vi "Shooter Loop.vi"(11 "Shooter Control":T2) -> (0 "Punch":T1, 1 "Trigger":T1, 2 "Release":T1, 3 "Add":T1, 5 "State":T4, 7 "Is Ready?":bool)   [LabVIEW 2013]
uses:
  <vilib>/Rock Robotics/WPI/Solenoid/WPI_SolenoidValue.ctl
  Common Code/Shooter State.ctl
  Shooter Manual Control.ctl
  Shooter Command.ctl
  Shooter Status.ctl
  Common Code/Change Detect Int.vi
  Common Code/Change Detect Boolean.vi
  Robot Global Data.vi
  <vilib>/Rock Robotics/WPI/DigitalInput/WPI_DigitalInputRefNum Registry Get.vi
  <vilib>/Rock Robotics/WPI/DigitalInput/WPI_DigitalInputGetValue.vi
panel:
  in  "Is Retracted":bool
  in  "Pressure":dbl
  in  "Line":dbl
  in  "Reset Time":dbl
  in  "Release Time":dbl
  # "Debug controls under this box"
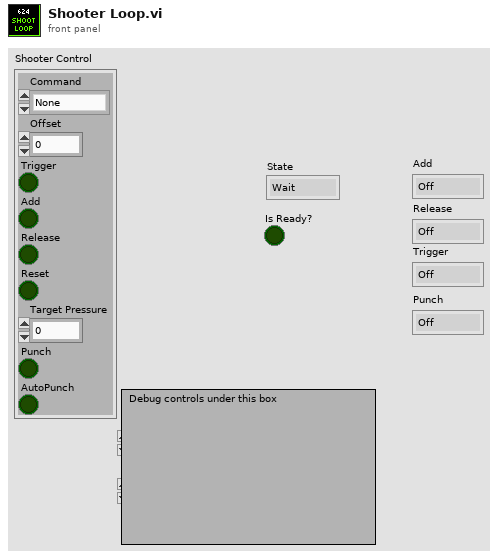
[diagram p1: front panel]
types:
  T1 = typedef "WPI_SolenoidValue.ctl" = enum16{"Off", "On", "Forward", "Reverse"}
  T2 = typedef "Shooter Manual Control.ctl" = cluster{"Command":T3, "Offset":dbl, "Trigger":bool, "Add":bool, "Release":bool, "Reset":bool, "Target Pressure":dbl, "Punch":bool, "AutoPunch":bool}
  T3 = typedef "Shooter Command.ctl" = enum16{"None", "Warmup", "Shoot", "Line Shoot", "Soft Shoot", "Toss"}
  T4 = typedef "Shooter State.ctl" = enum16{"Wait", "Fill Piston", "Lift Halo", "Trigger", "Reset", "Soft Release", "Soft Unpin", "Soft Refill", "Soft Shoot", "Toss Prep", "Toss Release"}
  T5 = typedef "Shooter Status.ctl" = cluster{"Shooter Ready":bool, "Add":bool, "Punch":bool, "Release":bool, "Trigger":bool, "High":bool, "State":T4}
  T6 = typedef "Dashboard UDP Packet.ctl" = cluster{"Camera":T7, "Gyro":T8, "Encoder":T10, "Auto Shift":T11, "Auton":T12, "Drive/Ramp X":dbl, "Drive/Ramp Y":dbl, "Drive/Battery Cutoff":dbl, "Pressure/Compressor Min Voltage":dbl, "Pressure/Compressor Delay":dbl, "Controller/Strafe Correction":bool, "Shooter":T13, "Rollers":T14, "Abort":bool, "Finish":bool, "IR Halo Sustain Time":dbl, "Disable Compressor":bool, "Center Omni Drive Delay":i32, "Vision Mode":T15, "Radius Throttle":bool, "Fieldcentric":T16, "Roll":T17, "Stick Deadband":dbl}
  T7 = typedef "Camera Controls.ctl" = cluster{"Camera/View Angle X":dbl, "Camera/Goal Track Timeout":dbl, "Camera/View Angle Y":dbl, "Camera/Goal Exposure":dbl, "Camera/Vision Receive Timeout":dbl, "Camera/Offset 1":dbl, "Camera/Offset 2":dbl}
  T8 = typedef "Gyro Controls.ctl" = cluster{"Gyro/Angle Tolerance":dbl, "Gyro/Steer Closeness Threshold":dbl, "Steer PID":T9, "Steer Close PID":T9}
  T9 = typedef "PID Params.ctl" = cluster{"max":dbl, "min":dbl, "P":dbl, "I":dbl, "D":dbl}
  T10 = typedef "Encoder Controls.ctl" = cluster{"Encoders/Reset":bool, "Encoders/Omni Constant":dbl, "Encoders/Omni Tick Constant":dbl, "Encoders/Left Constant":dbl, "Encoders/Right Constant":dbl, "Encoders/Right Tick Constant":dbl}
  T11 = typedef "Auto Shift Controls.ctl" = cluster{"AutoShift/Upshift Throttle Accel":dbl, "AutoShift/Speed Threshold":dbl, "AutoShift/Upshift Throttle":dbl, "AutoShift/Upshift Accel":dbl, "AutoShift/Downshift Accel":dbl, "AutoShift/Downshift Throttle":dbl, "AutoShift/Delay":dbl, "AutoShift/Enabled":bool}
  T12 = typedef "Auton Controls.ctl" = cluster{"Auton/Left Shoot X-Coord":dbl, "Auton/Right Shoot X-Coord":dbl, "DistDrive/Distance Stop Threshold":dbl, "DistDrive/Max Stop Speed":dbl, "Auton/Back Piston Time":dbl, "Auton/Manual Hot":bool, "Auton/Manual Hot Right":bool, "Default X PID":T9, "Default Y PID":T9, "Half Over Delay":dbl}
  T13 = typedef "Shooter Controls.ctl" = cluster{"Shooter/Reset Time":dbl, "Shooter/Release Delay":dbl, "Shooter/Pressure Steady Time":dbl, "Shooter/Misfire Delay":dbl, "Shooter/Ball Settle Time":dbl, "Shooter/Line IR Delay":dbl, "Pressure/Upper PSI Time":dbl, "Pressure/Lower PSI Time":dbl, "Shooter/Punch Delay":dbl, "Shooter/Target Pressure":dbl, "Pressure/Line B":dbl, "Pressure/Line M":dbl, "Pressure/Shooter M":dbl, "Pressure/Shooter B":dbl, "Halo Time":dbl, "Soft Release Delay":dbl, "Soft Unpin Delay":dbl, "Soft Shoot Delay":dbl, "Toss Release Time":dbl}
  T14 = typedef "Roller Controls.ctl" = cluster{"Roller/Load IRs Verify Time":dbl, "Roller/Center IR Latch Time":dbl, "Roller/Speed Front":dbl, "Roller/Speed Back":dbl, "Roller/Entry Timeout":dbl, "Roller/To Center Timeout":dbl, "Roller/Sustain Time":dbl, "Roller/Verify Center Time":dbl}
  T15 = typedef "Vision Mode.ctl" = enum16{"Normal", "Extreme Left", "Extreme Right"}
  T16 = typedef "Fieldcentric Controls.ctl" = cluster{"Relative Angle":bool, "Point Robot":bool, "X/Y ratio low":dbl, "Steering Gain":dbl, "Force Omni Down":bool, "Enable":bool, "X/Y ratio high":dbl}
  T17 = typedef "Roll Maneuver.ctl" = cluster{"X 1":dbl, "Y 1":dbl, "Y 2":dbl, "X 2":dbl, "Y 3":dbl, "X 3":dbl, "Time 1":i32, "Time 2":i32, "Time 3":i32, "Angle Start":dbl, "Angle End":dbl, "Angle Linearity":dbl}
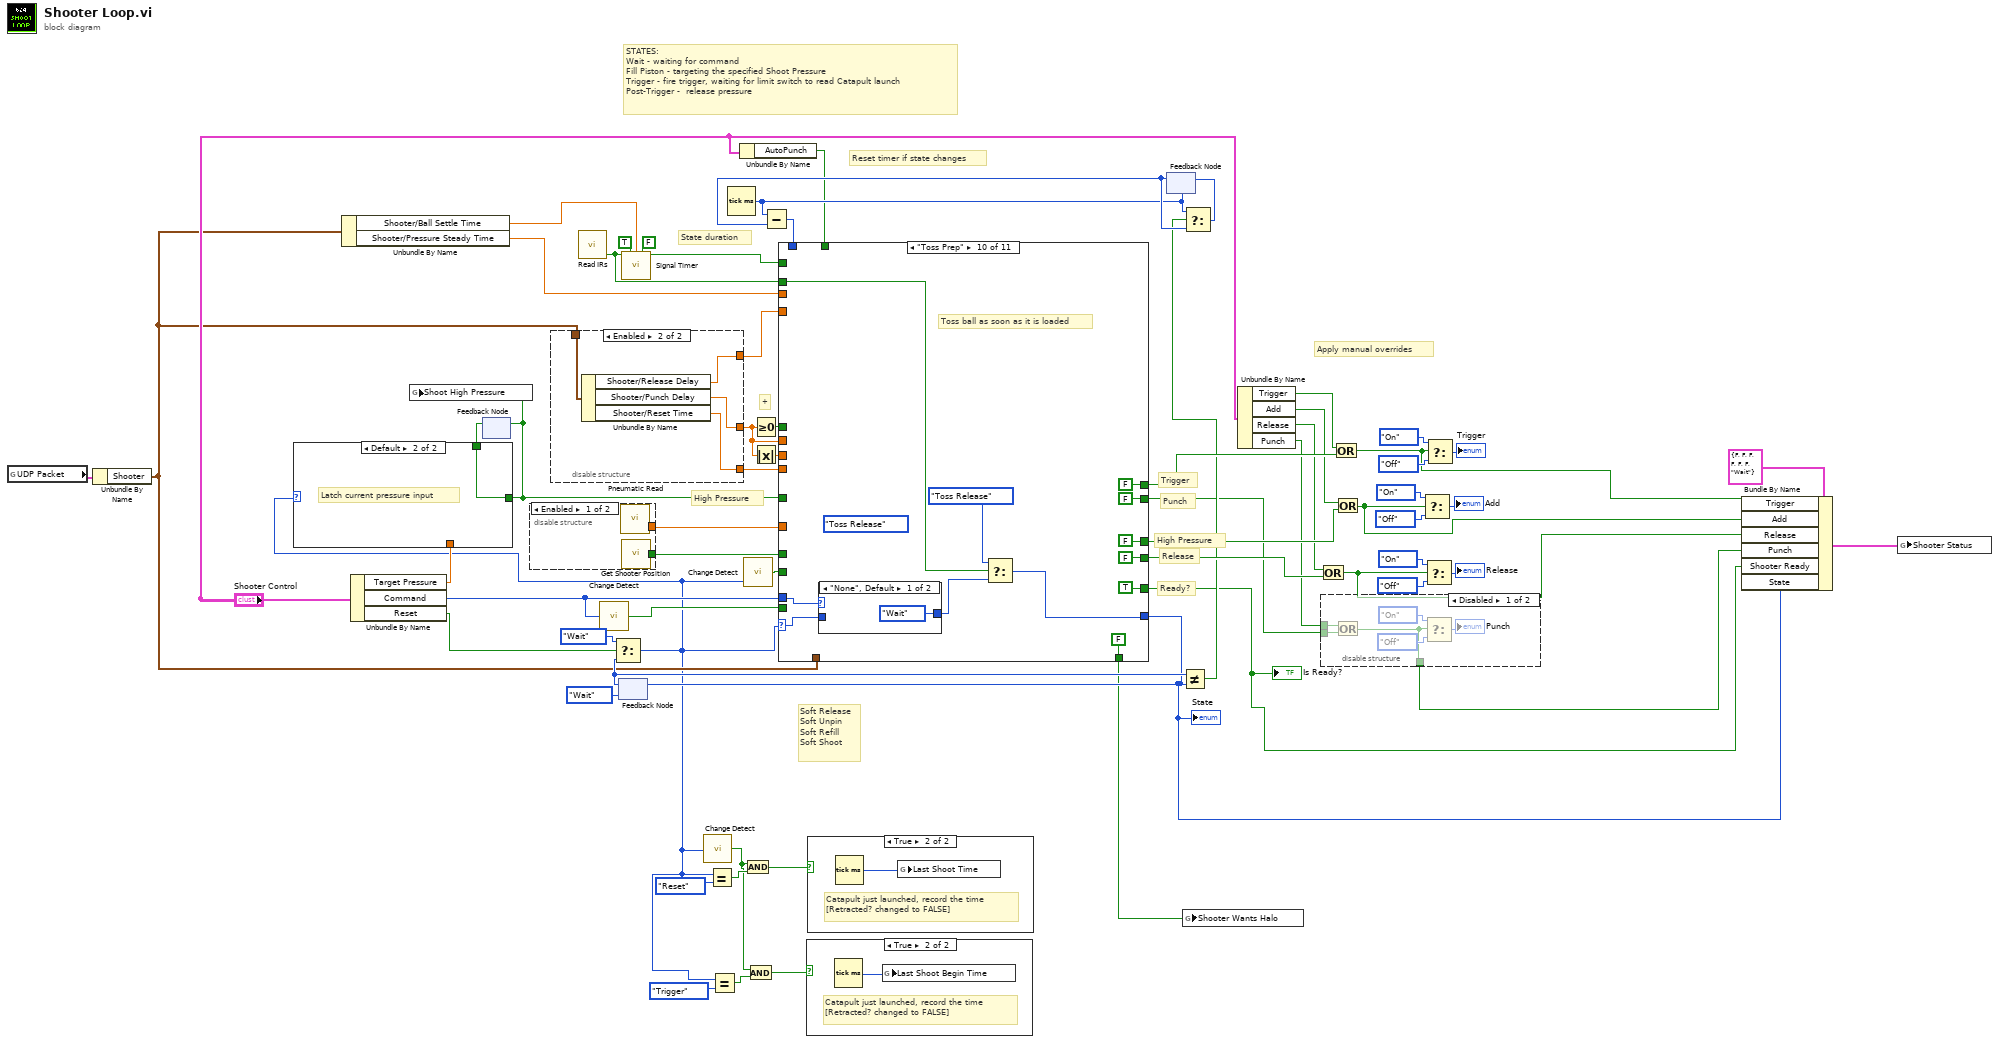
[diagram p0: block diagram]
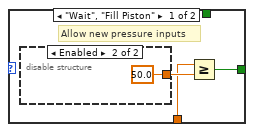
[diagram p4: hidden frame]
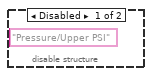
[diagram p5: hidden frame]
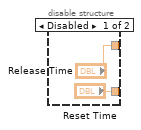
[diagram p7: hidden frame]
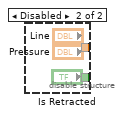
[diagram p8: hidden frame]
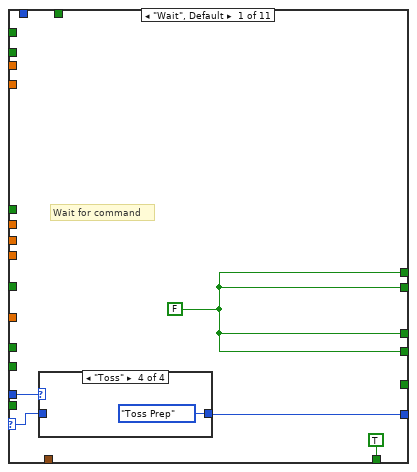
[diagram p9: hidden frame]
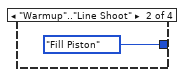
[diagram p11: hidden frame]
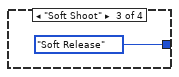
[diagram p12: hidden frame]
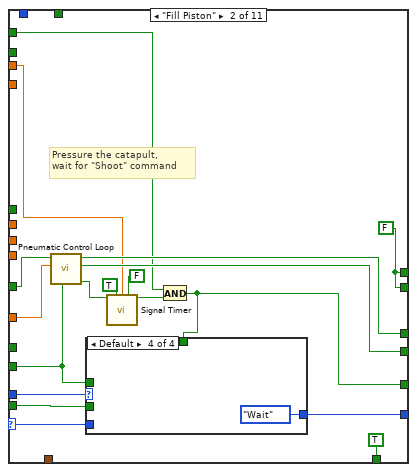
[diagram p13: hidden frame]
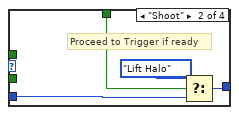
[diagram p15: hidden frame]
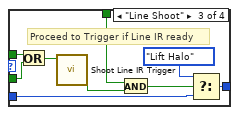
[diagram p16: hidden frame]
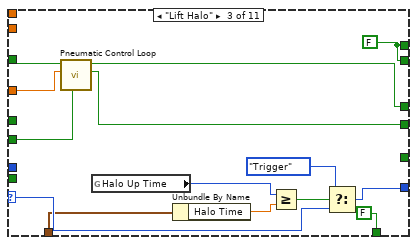
[diagram p17: hidden frame]
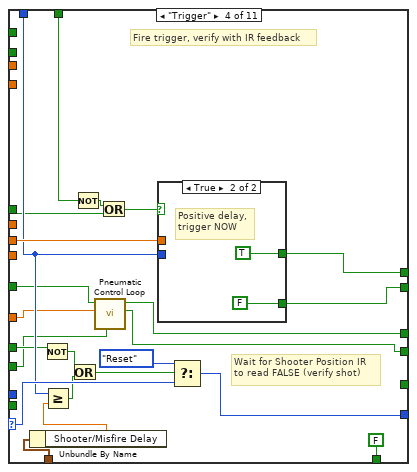
[diagram p18: hidden frame]
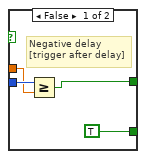
[diagram p19: hidden frame]
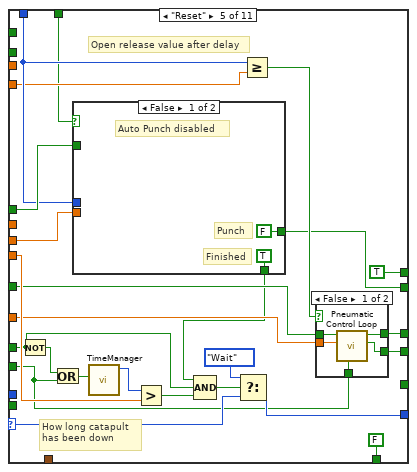
[diagram p20: hidden frame]
diagram:
  # "Soft Release\nSoft Unpin\nSoft Refill\nSoft Shoot"
  # "Punch"
  # "High Pressure"
  # "+"
  # "Apply manual overrides"
  # "Ready?"
  # "Release"
  # "High Pressure"
  # "Trigger"
  # "STATES:\nWait - waiting for command\nFill Piston - targeting the specified Shoot Pressure\nTrigger - fire trigger, waiting for limit switch to read Catapult launch\nPost-Trigger -  release pressure"
  # "State duration"
  # "Reset timer if state changes"
  n1 = global read "Robot Global Data.vi" "UDP Packet"() -> (w16:T6)
  n2 = Unbundle By Name(w16) -> ("Shooter"=w4:T13)
  n3 = Unbundle By Name(w4) -> ("Shooter/Ball Settle Time"=w15:dbl, "Shooter/Pressure Steady Time"=w14:dbl)
  n4 = Unbundle By Name("Shooter Control") -> ("Target Pressure"=w27:dbl, "Command"=w28:T3, "Reset"=w42:bool)
  n5 = feedback #1() -> (w26:bool)  [unwired: 1 in]
  n6 = disable-structure shown="Enabled" {
    disable-tunnel: [w68 "Pressure"] -> w65
    disable-tunnel: [w67 "Is Retracted"] -> w32
    frame Enabled {
      n7 = call "Pneumatic Read.vi"() -> ("Shooter"=w68:dbl)  [unwired: 2 in, 1 out]
      n8 = call "Get Shooter Position.vi"() -> ("Is Retracted"=w67:bool)  [unwired: 1 in]
    }
    frame Disabled {
    }
  }
  n9 = disable-structure shown="Enabled" {
    disable-tunnel: ["Reset Time" w73] -> w38
    disable-tunnel: ["Release Time" w74] -> w29
    disable-tunnel: [_ w75] -> w30
    disable-tunnel: w4 -> [_ w76]
    frame Disabled {
    }
    frame Enabled {
      n10 = Unbundle By Name(w76) -> ("Shooter/Release Delay"=w75:dbl, "Shooter/Punch Delay"=w74:dbl, "Shooter/Reset Time"=w73:dbl)
    }
  }
  n11 = call "Read IRs.vi"() -> ("Center"=w1:bool)  [unwired: 2 in, 3 out]
  n12 = call-poly "Change Detect.vi"("In"=w28) -> ("Changed?"=w3:bool)
  n13 = feedback #2(Shooter_State."Wait") -> (w43:T4)
  n14 = Select(t=Shooter_State."Wait", s=w42, f=w43) -> (s? t:f=w2:T4)
  n15 = case shown="Default" w2 {
    tunnel: w27 -> [w78 _]
    tunnel: [w77 w82] -> w21
    tunnel: w26 -> [_ w82]
    frame "Wait", "Fill Piston" {
      # "Allow new pressure inputs"
      n16 = disable-structure shown="Enabled" {
        disable-tunnel: [_ 50.0 ("Numeric")] -> w79
        frame Disabled {
          w80 = "Pressure/Upper PSI" ("Name")
        }
        frame Enabled {
        }
      }
      n17 = Greater Or Equal?(x=w78, y=w79) -> (x >= y?=w77:bool)
    }
    frame Default {
      # "Latch current pressure input"
    }
  }
  n18 = global write "Robot Global Data.vi" "Shoot High Pressure"(w21) -> ()
  n19 = feedback-in #1(w21) -> ()
  n20 = call "Signal Timer.vi"("Input"=w1, "Edge"=TRUE, "Interval"=w15, "Pull"=FALSE) -> ("Filtered Output"=w34:bool)  [unwired: 11 in]
  n21 = call-poly "Change Detect.vi"("In"=w2) -> ("Changed?"=w18:bool)
  n22 = Equal?(x=w2, y=Shooter_State."Reset") -> (x = y?=w33:bool)
  n23 = Equal?(x=w2, y=Shooter_State."Trigger") -> (x = y?=w19:bool)
  n24 = Tick Count (ms)() -> (millisecond timer value=w61:u32)
  n25 = Unbundle By Name("Shooter Control") -> ("AutoPunch"=w22:bool)
  n26 = call-poly "Change Detect.vi"("In"=w2) -> ("Changed?"=w37:bool)
  n27 = And(x=w18, y=w33) -> (x .and. y?=w41:bool)
  n28 = And(x=w18, y=w19) -> (x .and. y?=w17:bool)
  n29 = Greater Or Equal To 0?(x=w29) -> (x >= 0?=w40:bool)
  n30 = Absolute Value(x=w29) -> (abs(x)=w39:dbl)
  n31 = case shown="True" w17 {
    frame False {
    }
    frame True {
      # "Catapult just launched, record the time\n[Retracted? changed to FALSE]"
      n32 = Tick Count (ms)() -> (millisecond timer value=w83:u32)
      n33 = global write "Robot Global Data.vi" "Last Shoot Begin Time"(w83) -> ()
    }
  }
  n34 = case shown="True" w41 {
    frame False {
    }
    frame True {
      # "Catapult just launched, record the time\n[Retracted? changed to FALSE]"
      n35 = Tick Count (ms)() -> (millisecond timer value=w84:u32)
      n36 = global write "Robot Global Data.vi" "Last Shoot Time"(w84) -> ()
    }
  }
  n37 = feedback #3(w61) -> (w63:u32)
  n38 = Subtract(x=w61, y=w63) -> (x-y=w62:u32)
  n39 = case shown="\"Toss Prep\"" w2 {
    selector: w2 -> [w87 w106 w131 w163 w194 w213 w232 w245 w254 w267 w285]
    tunnel: [w88 w107 w129 w162 w193 w214 w233 w246 w255 w265 w283] -> w7
    tunnel: [w86 w111 w136 w149 w186 FALSE ("Finished") FALSE ("Finished") FALSE ("Finished") FALSE ("Finished") FALSE ("Finished") FALSE ("Finished")] -> w49
    tunnel: [w86 w110 w137 w148 w185 TRUE ("Release") TRUE ("Release") FALSE ("Release") FALSE ("Release") FALSE ("Release") TRUE ("Release")] -> w47
    tunnel: w65 -> [_ w109 w139 w152 w183 _ _ _ _ _ _]
    tunnel: w32 -> [_ _ _ w157 w176 _ _ w242 _ _ _]
    tunnel: w28 -> [w89 w108 _ _ _ w215 _ _ _ w268 _]
    tunnel: [_ w99 _ _ _ w212 _ _ _ TRUE _] -> w8
    tunnel: w62 -> [_ _ _ w158 w181 w216 w234 _ w256 _ _]
    tunnel: w39 -> [_ _ _ w160 w191 _ _ _ _ _ _]
    tunnel: [w86 w95 w135 w159 TRUE ("Trigger") FALSE ("Trigger") TRUE ("Trigger") TRUE ("Trigger") TRUE ("Trigger") FALSE ("Trigger") FALSE ("Trigger")] -> w51
    tunnel: w40 -> [_ _ _ w147 w192 _ _ _ _ _ _]
    tunnel: w38 -> [_ _ _ _ w187 _ _ _ _ _ _]
    tunnel: w37 -> [_ w98 w138 w151 w178 _ _ _ _ _ w289]
    tunnel: w14 -> [_ w101 _ _ _ _ _ _ _ _ _]
    tunnel: w34 -> [_ w100 _ _ _ _ _ _ _ _ _]
    tunnel: w30 -> [_ _ _ _ w180 _ _ _ _ _ _]
    tunnel: w29 -> [_ _ _ _ _ _ _ _ _ _ _]
    tunnel: w3 -> [_ w97 _ _ _ _ _ _ _ _ _]
    tunnel: w21 -> [_ w96 w140 w153 w184 _ _ _ _ _ _]
    tunnel: [w86 w95 w135 w150 w175 FALSE ("Finished") FALSE ("Finished") FALSE ("Finished") FALSE ("Finished") FALSE ("Finished") FALSE ("Finished")] -> w24
    tunnel: w22 -> [_ _ _ w145 w172 _ _ _ _ _ _]
    tunnel: [TRUE ("Trigger") TRUE ("Trigger") FALSE ("Trigger") FALSE ("Trigger") FALSE ("Trigger") TRUE ("Trigger") FALSE ("Trigger") FALSE ("Trigger") FALSE ("Trigger") FALSE ("Trigger") FALSE ("Trigger")] -> w6
    tunnel: w4 -> [_ _ w127 w141 _ w218 w236 _ w258 _ w290]
    tunnel: w1 -> [_ _ _ _ _ _ _ _ _ w264 _]
    frame "Wait", Default {
      w86 = FALSE ("Finished")
      # "Wait for command"
      n40 = case shown="\"Toss\"" w89 {
        tunnel: [w90 Shooter_State."Fill Piston" ("t") Shooter_State."Soft Release" ("t") Shooter_State."Toss Prep" ("t")] -> w88
        tunnel: w87 -> [w90 _ _ _]
        frame Default {
        }
        frame "Warmup".."Line Shoot" {
        }
        frame "Soft Shoot" {
        }
        frame "Toss" {
        }
      }
    }
    frame "Fill Piston" {
      w95 = FALSE ("Finished")
      # "Pressure the catapult,\nwait for \"Shoot\" command"
      n41 = call "Pneumatic Control Loop.vi"("reinit"=w98, "Process Variable"=w109, "High Pressure"=w96) -> ("Finished"=w103:bool, "Release"=w110:bool, "High Pressure"=w111:bool)  [unwired: 6 in]
      n42 = call "Signal Timer.vi"("Input"=w103, "Edge"=TRUE, "Interval"=w101, "Pull"=FALSE) -> ("Filtered Output"=w102:bool)  [unwired: 11 in]
      n43 = And(x=w100, y=w102) -> (x .and. y?=w99:bool)
      n44 = case shown="Default" w108 {
        tunnel: [w112 w116 w125 Shooter_State."Wait" ("t")] -> w107
        tunnel: w106 -> [w112 w114 w123 _]
        tunnel: w99 -> [_ w113 w122 _]
        tunnel: w98 -> [_ _ w120 _]
        tunnel: w97 -> [_ _ w119 _]
        frame "None", "Warmup" {
          # "Wait for \"Shoot\" cmd"
        }
        frame "Shoot" {
          # "Proceed to Trigger if ready"
          n45 = Select(t=Shooter_State."Lift Halo", s=w113, f=w114) -> (s? t:f=w116:T4)
        }
        frame "Line Shoot" {
          # "Proceed to Trigger if Line IR ready"
          n46 = Or(x=w120, y=w119) -> (x .or. y?=w118:bool)
          n47 = call "Shoot Line IR Trigger.vi"("Reinit"=w118) -> ("Trigger"=w117:bool)  [unwired: 10 in]
          n48 = And(x=w122, y=w117) -> (x .and. y?=w121:bool)
          n49 = Select(t=Shooter_State."Lift Halo", s=w121, f=w123) -> (s? t:f=w125:T4)
        }
        frame Default {
        }
      }
    }
    frame "Lift Halo" {
      w135 = FALSE ("Trigger")
      n50 = call "Pneumatic Control Loop.vi"("reinit"=w138, "Process Variable"=w139, "High Pressure"=w140) -> ("Release"=w137:bool, "High Pressure"=w136:bool)  [unwired: 6 in, 1 out]
      n51 = global read "Robot Global Data.vi" "Halo Up Time"() -> (w134:i32)
      n52 = Unbundle By Name(w127) -> ("Halo Time"=w133:dbl)
      n53 = Greater Or Equal?(x=w134, y=w133) -> (x >= y?=w132:bool)
      n54 = Select(t=Shooter_State."Trigger", s=w132, f=w131) -> (s? t:f=w129:T4)
    }
    frame "Trigger" {
      # "Fire trigger, verify with IR feedback"
      # "Wait for Shooter Position IR\nto read FALSE (verify shot)"
      n55 = Unbundle By Name(w141) -> ("Shooter/Misfire Delay"=w142:dbl)
      n56 = Not(x=w157) -> (.not. x?=w156:bool)
      n57 = Greater Or Equal?(x=w158, y=w142) -> (x >= y?=w155:bool)
      n58 = Or(x=w156, y=w155) -> (x .or. y?=w154:bool)
      n59 = Not(x=w145) -> (.not. x?=w146:bool)
      n60 = call "Pneumatic Control Loop.vi"("reinit"=w151, "Process Variable"=w152, "High Pressure"=w153) -> ("Release"=w148:bool, "High Pressure"=w149:bool)  [unwired: 6 in, 1 out]
      n61 = Or(x=w146, y=w147) -> (x .or. y?=w144:bool)
      n62 = case shown="True" w144 {
        tunnel: w158 -> [w166 _]
        tunnel: w160 -> [w165 _]
        tunnel: [w164 TRUE ("Finished")] -> w159
        tunnel: [TRUE ("Finished") FALSE ("Finished")] -> w150
        frame False {
          # "Negative delay\n[trigger after delay]"
          n63 = Greater Or Equal?(x=w166, y=w165) -> (x >= y?=w164:bool)
        }
        frame True {
          # "Positive delay,\ntrigger NOW"
        }
      }
      n64 = Select(t=Shooter_State."Reset", s=w154, f=w163) -> (s? t:f=w162:T4)
    }
    frame "Reset" {
      # "How long catapult\nhas been down"
      # "Open release value after delay"
      n65 = Not(x=w176) -> (.not. x?=w182:bool)
      n66 = Or(x=w182, y=w178) -> (x .or. y?=w188:bool)
      n67 = case shown="False" w172 {
        tunnel: w192 -> [_ w200]
        tunnel: w191 -> [_ w199]
        tunnel: w181 -> [_ w198]
        tunnel: [FALSE w197] -> w175
        tunnel: [TRUE w197] -> w173
        frame False {
          # "Punch"
          # "Finished"
          # "Auto Punch disabled"
        }
        frame True {
          n68 = case shown="True" w200 {
            tunnel: w198 -> [_ w204]
            tunnel: w199 -> [_ w203]
            tunnel: [TRUE w202] -> w197
            frame False {
              # "Negative delay\n[punch already started\nin \"Trigger\" state]"
            }
            frame True {
              # "Positive delay\n[release after delay]"
              n69 = Greater Or Equal?(x=w204, y=w203) -> (x >= y?=w202:bool)
            }
          }
        }
      }
      n70 = call "TimeManager.vi"("Reset?"=w188) -> ("Time Since Reset"=w189:u32)  [unwired: 9 in, 1 out]
      n71 = Greater?(x=w189, y=w187) -> (0:w177:bool)
      n72 = Compound Arithmetic op=AND(w173, w176, w177) -> (w174:bool)
      n73 = Select(t=Shooter_State."Wait", s=w174, f=w194) -> (s? t:f=w193:T4)
      n74 = Greater Or Equal?(x=w181, y=w180) -> (x >= y?=w179:bool)
      n75 = case shown="False" w179 {
        tunnel: [w209 FALSE ("Finished")] -> w186
        tunnel: [w208 TRUE ("Release")] -> w185
        tunnel: w184 -> [w207 _]
        tunnel: w183 -> [w206 _]
        tunnel: w178 -> [w205 _]
        frame False {
          n76 = call "Pneumatic Control Loop.vi"("reinit"=w205, "Process Variable"=w206, "High Pressure"=w207) -> ("Release"=w208:bool, "High Pressure"=w209:bool)  [unwired: 6 in, 1 out]
        }
        frame True {
          # "Release"
        }
      }
    }
    frame "Soft Release" {
      # "Dump all pressure"
      n77 = Unbundle By Name(w218) -> ("Soft Release Delay"=w217:dbl)
      n78 = Greater Or Equal?(x=w216, y=w217) -> (x >= y?=w212:bool)
      n79 = case shown="\"Shoot\"" w215 {
        tunnel: [Shooter_State."Wait" ("t") w225 w228] -> w214
        tunnel: w213 -> [_ w225 w229]
        tunnel: w212 -> [_ _ w227]
        frame Default {
          # "Other command, return to \"Wait\"\n(safe to abandon \"soft\" mode)"
        }
        frame "None", "Soft Shoot" {
          # "Wait for \"Shoot\" command"
        }
        frame "Shoot" {
          # "If pressure released, continue to unpin"
          n80 = Select(t=Shooter_State."Soft Unpin", s=w227, f=w229) -> (s? t:f=w228:T4)
        }
      }
    }
    frame "Soft Unpin" {
      # "Unpin the Trigger \n(for X ms)"
      # "After delay, proceed to Refill"
      n81 = Unbundle By Name(w236) -> ("Soft Unpin Delay"=w235:dbl)
      n82 = Greater Or Equal?(x=w234, y=w235) -> (x >= y?=w231:bool)
      n83 = Select(t=Shooter_State."Soft Refill", s=w231, f=w232) -> (s? t:f=w233:T4)
    }
    frame "Soft Refill" {
      # "Re-add pressure\n(start timer after Limit Switch releases)"
      # "Re-add\npressure"
      # "After shooter deploys,\nproceed to Soft Shoot"
      n84 = Not(x=w242) -> (.not. x?=w243:bool)
      n85 = Select(t=Shooter_State."Soft Shoot", s=w243, f=w245) -> (s? t:f=w246:T4)
    }
    frame "Soft Shoot" {
      # "Re-add\npressure"
      # "After delay, proceed to Reset"
      n86 = Unbundle By Name(w258) -> ("Soft Shoot Delay"=w257:dbl)
      n87 = Greater Or Equal?(x=w256, y=w257) -> (x >= y?=w253:bool)
      n88 = Select(t=Shooter_State."Reset", s=w253, f=w254) -> (s? t:f=w255:T4)
    }
    frame "Toss Prep" {
      (unwired) Shooter_State."Toss Release" ("t")
      # "Toss ball as soon as it is loaded"
      n89 = case shown="\"None\", Default" w268 {
        tunnel: w267 -> [_ w277]
        tunnel: [Shooter_State."Wait" ("t") w277] -> w266
        frame "None", Default {
        }
        frame "Toss" {
        }
      }
      n90 = Select(t=Shooter_State."Toss Release", s=w264, f=w266) -> (s? t:f=w265:T4)
    }
    frame "Toss Release" {
      # "Just use unpin cases, we \ndon't need any special new ones\n(lazy)"
      # "Release air for the specified time\nto lower shooter power"
      n91 = Unbundle By Name(w290) -> ("Toss Release Time"=w287:dbl)
      n92 = call "TimeManager.vi"("Reset?"=w289) -> ("Time Since Reset"=w288:u32)  [unwired: 9 in, 1 out]
      n93 = Greater Or Equal?(x=w288, y=w287) -> (x >= y?=w286:bool)
      n94 = Select(t=Shooter_State."Soft Unpin", s=w286, f=w285) -> (s? t:f=w283:T4)
    }
  }
  "State" <- w7
  "Is Ready?" <- w8
  n95 = feedback-in #2(w7) -> ()
  n96 = Not Equal?(x=w43, y=w7) -> (x != y?=w45:bool)
  n97 = global write "Robot Global Data.vi" "Shooter Wants Halo"(w6) -> ()
  n98 = Select(t=w61, s=w45, f=w63) -> (s? t:f=w64:u32)
  n99 = feedback-in #3(w64) -> ()
  n100 = Unbundle By Name("Shooter Control") -> ("Trigger"=w50:bool, "Add"=w48:bool, "Release"=w46:bool, "Punch"=w25:bool)
  n101 = Or(x=w46, y=w47) -> (x .or. y?=w10:bool)
  n102 = disable-structure shown="Disabled" {
    disable-tunnel: w25 -> [w293 _]
    disable-tunnel: w24 -> [w292 _]
    disable-tunnel: [w291 _] -> w9
    frame Disabled {
      n103 = Or(x=w293, y=w292) -> (x .or. y?=w291:bool)
      n104 = Select(t=WPI_SolenoidValue."On" ("Solenoid Output"), s=w291, f=WPI_SolenoidValue."Off" ("Solenoid Output")) -> (s? t:f=→"Punch":T1)
    }
    frame Enabled {
    }
  }
  n105 = Or(x=w50, y=w51) -> (x .or. y?=w12:bool)
  n106 = Or(x=w48, y=w49) -> (x .or. y?=w11:bool)
  n107 = Select(t=WPI_SolenoidValue."On" ("Solenoid Output"), s=w11, f=WPI_SolenoidValue."Off" ("Solenoid Output")) -> (s? t:f=→"Add":T1)
  n108 = Select(t=WPI_SolenoidValue."On" ("Solenoid Output"), s=w10, f=WPI_SolenoidValue."Off" ("Solenoid Output")) -> (s? t:f=→"Release":T1)
  n109 = Select(t=WPI_SolenoidValue."On" ("Solenoid Output"), s=w12, f=WPI_SolenoidValue."Off" ("Solenoid Output")) -> (s? t:f=→"Trigger":T1)
  n110 = Bundle By Name(cluster=T5 {"Shooter Ready"=FALSE, "Add"=FALSE, "Punch"=FALSE, "Release"=FALSE, "Trigger"=FALSE, "High"=FALSE, "State"=enum."Wait"} ("Shooter Status"), "Trigger"=w12, "Add"=w11, "Release"=w10, "Punch"=w9, "Shooter Ready"=w8, "State"=w7) -> (w5:T5)
  n111 = global write "Robot Global Data.vi" "Shooter Status"(w5) -> ()
